vi "TDMSAdv open.vi"(7 "file format version":enum16{"1.0", "2.0", "Adv"}(ring)=enum."Adv", 8 "error in (no error)":errorcluster, 9 "operation (0:open)":T1(ring), 10 "openPath":path, 11 "TDMSAdv in":refnum<class "TDMSAdv.lvclass">) -> (0 "error out":errorcluster, 3 "TDMSAdv out":refnum<class "TDMSAdv.lvclass">)   [LabVIEW 2018, in "TDMSAdv.lvclass"]
uses:
  TDMSAdv.lvclass
  TDMSAdv.lvclass/TDMSAdv.ctl
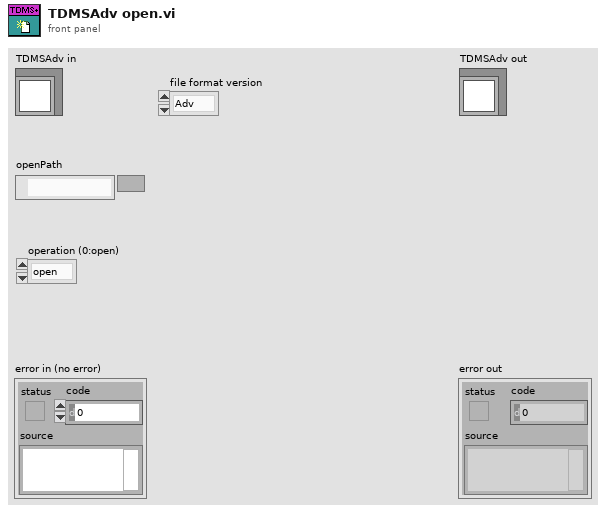
[diagram p1: front panel]
types:
  T1 = enum16{"open", "open or create", "create or replace", "create", "open (read-only)"}
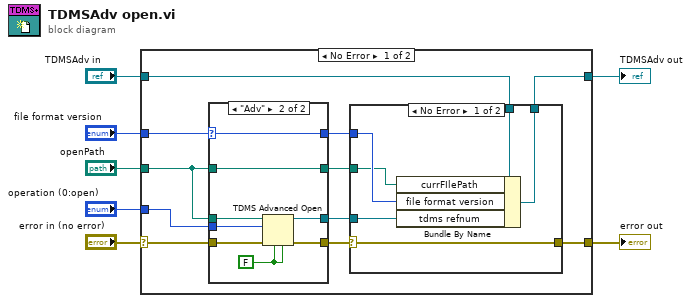
[diagram p0: block diagram]
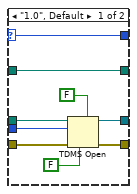
[diagram p2: hidden frame]
diagram:
  n1 = case shown="No Error" "error in (no error)" {
    selector: "error in (no error)" -> [w17 w45]
    tunnel: [w13 w45] -> w6
    tunnel: [w16 w44] -> w4
    tunnel: "TDMSAdv in" -> [w12 w44]
    tunnel: "openPath" -> [w9 _]
    tunnel: "operation (0:open)" -> [w18 _]
    tunnel: "file format version" -> [w11 _]
    frame No Error {
      n2 = case shown="\"Adv\"" w11 {
        selector: w11 -> [w22 w29]
        tunnel: w18 -> [w26 w35]
        tunnel: w17 -> [w25 w34]
        tunnel: [w23 w32] -> w15
        tunnel: [w24 w31] -> w14
        tunnel: w9 -> [w27 w30]
        tunnel: [w22 w29] -> w10
        tunnel: w9 -> [w19 w28]
        tunnel: [w19 w28] -> w8
        frame "1.0", Default {
          n3 = TDMS Open(5:FALSE ("create index file? (T)"), 6:FALSE ("disable buffering? (T)"), 8:w25, 10:w26, 11:w27) -> (0:w24:errorcluster, 3:w23:refnum<k34>)  [unwired: 2 in]
        }
        frame "Adv" {
          w33 = FALSE ("disable buffering? (T)")
          n4 = TDMS Advanced Open(4:w33, 6:w33, 8:w34, 10:w35, 11:w30) -> (0:w31:errorcluster, 3:w32:refnum<k34>)  [unwired: 1 out]
        }
      }
      n5 = case shown="No Error" w14 {
        selector: w14 -> [w38 w42]
        tunnel: w12 -> [w41 w43]
        tunnel: [w40 w43] -> w16
        tunnel: w15 -> [w39 _]
        tunnel: [w38 w42] -> w13
        tunnel: w10 -> [w37 _]
        tunnel: w8 -> [w36 _]
        frame No Error {
          n6 = Bundle By Name(cluster=w41, "currFIlePath"=w36, "file format version"=w37, "tdms refnum"=w39) -> (w40:refnum<class "TDMSAdv.lvclass">)
        }
        frame Error {
        }
      }
    }
    frame Error {
    }
  }
  "error out" <- w6
  "TDMSAdv out" <- w4
